vi "Open Selected Preset SubVI.vi"(8 "error in (no error)":errorcluster, 9 "Controls":refnum<vi>[](array[refnum]), 10 "Current Preset":string, 11 "Preset Directory:":path) -> (0 "error out":errorcluster)   [LabVIEW 2018]
uses:
  Load and Save Controls_LV2009.llb/RWC_Actions.ctl
  <vilib>/Utility/config.llb/NI_LVConfig.lvlib
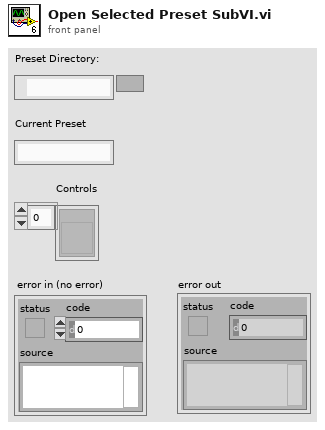
[diagram p1: front panel]
types:
  T1 = typedef "RWC_Actions.ctl" = enum16{"Read", "Write", "Read and Create"}
  T2 = typedef "NI_LVConfig.lvlib/Config Data RefNum.ctl" = refnum<k1>
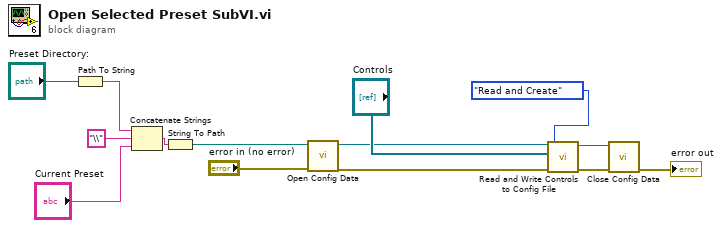
[diagram p0: block diagram]
diagram:
  n1 = Path To String(path="Preset Directory:") -> (string=w9:string)
  n2 = Concatenate Strings(w9, "\\", "Current Preset") -> (w1:string)
  n3 = String To Path(string=w1) -> (path=w8:path)
  n4 = call <vilib>:"Open Config Data.vi"("error in (no error)"="error in (no error)", "configuration file path"=w8) -> ("error out"=w4:errorcluster, "refnum"=w7:T2)  [unwired: 7 in, 1 out]
  n5 = call "Read and Write Controls to Config File.vi"("Action"=RWC_Actions."Read and Create", "error in"=w4, "Control References"="Controls", "Configuration File Reference In"=w7) -> ("error out"=w3:errorcluster, "Configuration File Reference Out"=w6:T2)  [unwired: 6 in]
  n6 = call <vilib>:"Close Config Data.vi"("error in (no error)"=w3, "refnum"=w6) -> ("error out"=→"error out":errorcluster)  [unwired: 8 in, 1 out]
